vi "find or create references.vi"(6 "application reference (local)":refnum<vi>, 7 "vi type":T1, 8 "Data Interface VI":string, 9 "index ctl":string, 10 "data ctl":string, 11 "runtime":refnum<vi>) -> (0 "error out":errorcluster, 3 "vi refs":T2)   [LabVIEW 2013, in "control module data interface generator.lvlib"]
uses:
  control module data interface generator.lvlib
  Controls/initialized references.ctl
  Controls/interface VI type.ctl
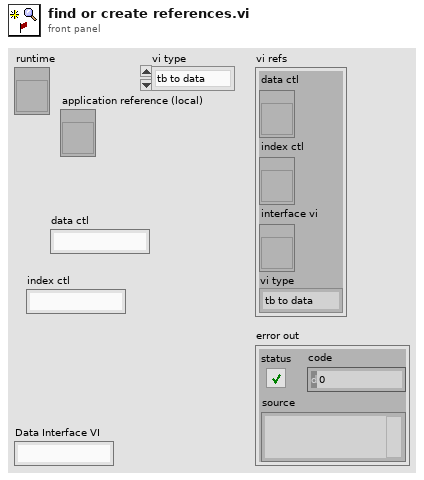
[diagram p1: front panel]
types:
  T1 = typedef "control module data interface generator.lvlib/interface VI type.ctl" = enum16{"tb to data", "data to tb"}
  T2 = typedef "control module data interface generator.lvlib/initialized references.ctl" = cluster{"data ctl":refnum<vi>, "index ctl":refnum<vi>, "interface vi":refnum<vi>, "vi type":T1}
  T3 = enum32{"invalid VI type", "Standard VI", "Control VI", "Global VI", "Polymorphic VI", "Configuration VI", "SubSystem", "Facade VI", "Method VI"}
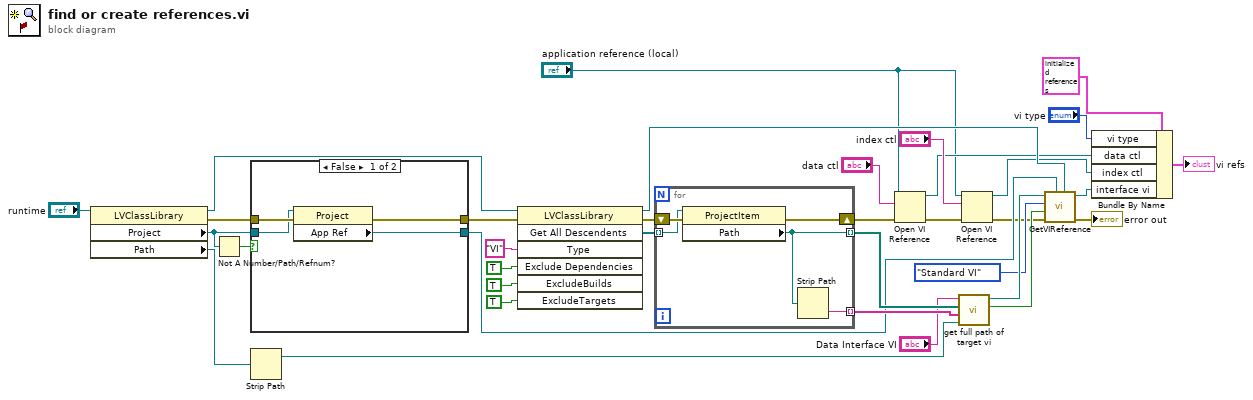
[diagram p0: block diagram]
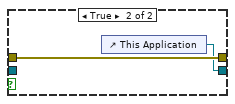
[diagram p2: hidden frame]
diagram:
  n1 = property class="LVClassLibrary"(reference="runtime") -> (reference out=w25:refnum<vi>, error out=w24:errorcluster, "Project"=w22:refnum<vi>, "Path"=w20:path)  [unwired: 1 in]
  n2 = Not A Number/Path/Refnum?(number/path/refnum=w22) -> (NaN/Path/Refnum?=w21:bool)
  n3 = case shown="False" w21 {
    tunnel: w24 -> [w39 w41]
    tunnel: [w38 w41] -> w23
    tunnel: w22 -> [w37 _]
    tunnel: [w36 w40] -> w12
    frame False {
      n4 = property class="Project"(reference=w37, error in=w39) -> (error out=w38:errorcluster, "App Ref"=w36:refnum<vi>)  [unwired: 1 out]
    }
    frame True {
      n5 = control-ref of="This Application"() -> (w40:refnum<vi>)
    }
  }
  n6 = Strip Path(path=w20) -> (stripped path=w16:path)  [unwired: 1 out]
  n7 = invoke class="LVClassLibrary" method="Get All Descendents"(reference=w25, error in=w23, "Type"="VI", "Exclude Dependencies"=TRUE ("ExcludeDependencies"), "ExcludeBuilds"=TRUE, "ExcludeTargets"=TRUE) -> (reference out=w10:refnum<vi>, error out=w27:errorcluster, "All Descendents"=w26:refnum<vi>[])  [unwired: 1 in, 4 out]
  n8 = for {
    shift-right: [w44] -> w2
    shift-left: w27 -> [w46]
    tunnel: w26 -> [w45] mode=indexing
    tunnel: [w43] -> w19 mode=indexing
    tunnel: [w42] -> w18 mode=indexing
    n9 = property class="ProjectItem"(reference=w45, error in=w46) -> (error out=w44:errorcluster, "Path"=w43:path)  [unwired: 1 out]
    n10 = Strip Path(path=w43) -> (name=w42:string)  [unwired: 1 out]
  }
  n11 = Open VI Reference(application reference (local)="application reference (local)", vi path="data ctl", error in (no error)=w2) -> (vi reference=w3:refnum<vi>, error out=w7:errorcluster)  [unwired: 3 in]
  n12 = call "get full path of target vi.vi"("class folder path"=w16, "class vi names"=w18, "class vi paths"=w19, "vi to qualify"="Data Interface VI") -> ("not in class"=w9:bool, "full path"=w13:path)  [unwired: 6 in]
  n13 = Open VI Reference(application reference (local)="application reference (local)", vi path="index ctl", error in (no error)=w7) -> (vi reference=w4:refnum<vi>, error out=w8:errorcluster)  [unwired: 3 in]
  n14 = call "GetVIReference.vi"("LVClassLibrary in"=w10, "application reference"=w12, "error in"=w8, "not in class"=w9, "vi type"=T3."Standard VI", "file path"=w13) -> ("error out"=→"error out":errorcluster, "reference out"=w14:refnum<vi>)  [unwired: 4 in]
  n15 = Bundle By Name(cluster=T2 {"data ctl"=refnum, "index ctl"=refnum, "interface vi"=refnum, "vi type"=enum."tb to data"} ("vi refs"), "vi type"="vi type", "data ctl"=w3, "index ctl"=w4, "interface vi"=w14) -> (→"vi refs":T2)
